vi "oauth2_token_pkce.vi"(6 "redirect_uri":string, 8 "error in (no error)":errorcluster, 9 "code_verifier":string, 10 "client_id":string, 11 "authorization_code":string) -> (0 "error out":errorcluster, 3 "access_token":string)   [LabVIEW 2015, in "lv-dropbox.lvlib"]
uses:
  lv-dropbox.lvlib
  private/_controls/content_type.ctl
  <vilib>/httpClient/POSTBuffer.vi
  <vilib>/httpClient/LabVIEWHTTPClient.lvlib
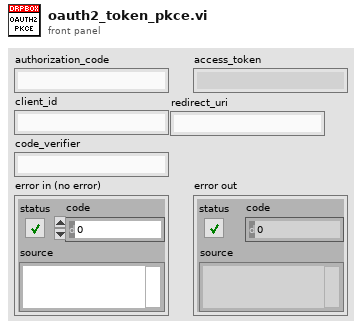
[diagram p1: front panel]
types:
  T1 = typedef "lv-dropbox.lvlib/content_type.ctl" = enum16{"<content_type>", "application/json", "application/octet-stream", "application/x-www-form-urlencoded"}
  T2 = cluster{"access_token":string, "expires_in":dbl, "token_type":string}
  T3 = typedef "LabVIEWHTTPClient.lvlib/ClientHandle.ctl" = refnum<k1>
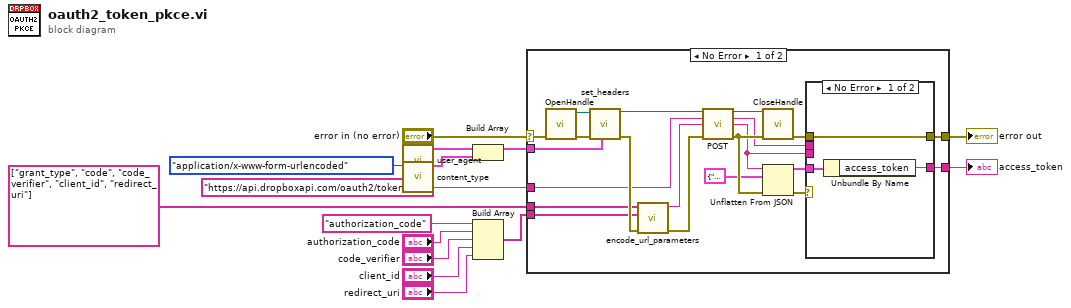
[diagram p0: block diagram]
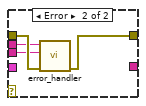
[diagram p2: hidden frame]
diagram:
  n1 = call "user_agent.vi"() -> ("header"=w12:cluster{"header":string, "value":string})  [unwired: 11 in]
  n2 = call "content_type.vi"("content_type"=content_type."application/x-www-form-urlencoded") -> ("header"=w14:cluster{"header":string, "value":string})  [unwired: 10 in]
  n3 = Build Array(w12, w14) -> (w11:cluster{"header":string, "value":string}[])
  n4 = Build Array("authorization_code", "authorization_code", "code_verifier", "client_id", "redirect_uri") -> (w4:string[])
  n5 = case shown="No Error" "error in (no error)" {
    selector: "error in (no error)" -> [w30 w44]
    tunnel: "https://api.dropboxapi.com/oauth2/token" ("url") -> [w34 _]
    tunnel: w11 -> [w28 _]
    tunnel: [w23 w44] -> w13
    tunnel: string[] ["grant_type", "code", "code_verifier", "client_id", "redirect_uri"] -> [w19 _]
    tunnel: [w20 _] -> w8
    tunnel: w4 -> [w18 _]
    frame No Error {
      n6 = call <vilib>:"OpenHandle.vi"("error in (no error)"=w30) -> ("client handle out"=w31:T3, "error out"=w29:errorcluster)  [unwired: 13 in]
      n7 = call "set_headers.vi"("header_value []"=w28, "error in (no error)"=w29, "client_handle in"=w31) -> ("error out"=w36:errorcluster, "client_handle out"=w27:T3)  [unwired: 7 in]
      n8 = call "encode_url_parameters.vi"("error in (no error)"=w36, "value []"=w18, "key []"=w19) -> ("error out"=w16:errorcluster, "url_encoded_string"=w17:string)  [unwired: 7 in]
      n9 = call-poly <vilib>:"POST.vi"("client handle"=w27, "url"=w34, "buffer"=w17, "error in (no error)"=w16) -> ("client handle out"=w26:T3, "headers"=w22:string, "body"=w21:string, "error out"=w35:errorcluster)  [unwired: 8 in]
      n10 = call <vilib>:"CloseHandle.vi"("client handle"=w26, "error in (no error)"=w35) -> ("error out"=w24:errorcluster)  [unwired: 13 in]
      n11 = Unflatten From JSON(JSON string=w21, type and defaults=T2 {"access_token"="", "expires_in"=0.0, "token_type"=""} ("value"), error in (no error)=w35) -> (value=w32:T2, error out=w25:errorcluster)  [unwired: 4 in]
      n12 = case shown="No Error" w25 {
        tunnel: w32 -> [w38 _]
        tunnel: w24 -> [w39 w43]
        tunnel: [w39 w40] -> w23
        tunnel: w22 -> [_ w42]
        tunnel: w21 -> [_ w41]
        tunnel: [w37 _] -> w20
        frame No Error {
          n13 = Unbundle By Name(w38) -> ("access_token"=w37:string)
        }
        frame Error {
          n14 = call "error_handler.vi"("error in (no error)"=w43, "body"=w41, "headers"=w42) -> ("error out"=w40:errorcluster)  [unwired: 8 in]
        }
      }
    }
    frame Error {
    }
  }
  "error out" <- w13
  "access_token" <- w8
